vi "PID (DBL) Obsolete.vi"(6 "reinitialize? (F)":bool, 7 "output range":cluster{"output high":dbl, "output low":dbl}={"output high"=100.0, "output low"=-100.0} {"output low" format="%.2f"; "output high" format="%.2f"}, 8 "dt (s)":dbl=-1.0 format="%.3f", 9 "PID gains":T1={"proportional gain (Kc)"=1.0, "integral time (Ti, min)"=0.01, "derivative time (Td, min)"=0.0} {"derivative time (Td, min)" format="%.3f"; "integral time (Ti, min)" format="%.3f"; "proportional gain (Kc)" format="%.3f"}, 10 "process variable":dbl format="%.2f", 11 "setpoint":dbl format="%.2f") -> (0 "dt out (s)":dbl format="%.3f", 3 "output":dbl format="%.2f")   [LabVIEW 2020, in "NI_PID_pid.lvlib"]
doc: "PID algorithm for simple PID applications or high speed control applications that require an efficient algorithm. PID algorithm features control output range limiting with integrator anti-windup and bumpless controller output for PID gain changes."
uses:
  <vilib>/addons/control/pid/NI_PID_pid.lvlib
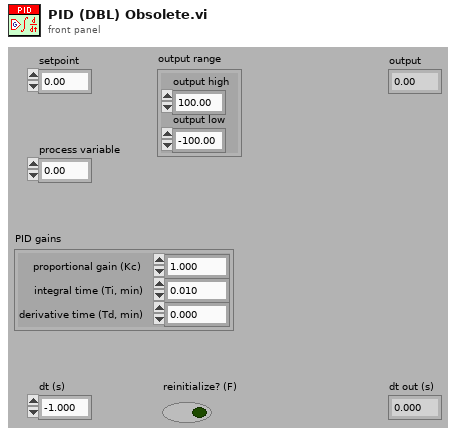
[diagram p1: front panel]
types:
  T1 = cluster{"proportional gain (Kc)":dbl, "integral time (Ti, min)":dbl, "derivative time (Td, min)":dbl}
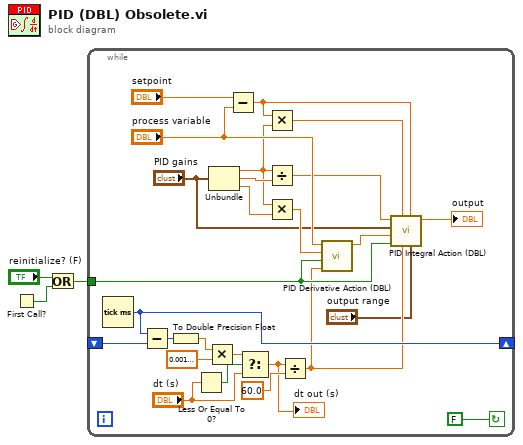
[diagram p0: block diagram]
diagram:
  n1 = First Call?() -> (First Call?: T/F=w3:bool)
  n2 = Or(x="reinitialize? (F)", y=w3) -> (x .or. y?=w2:bool)
  n3 = while {
    tunnel: w2 -> [w9]
    shift-left: _ -> [w23]
    shift-right: [w22] -> _
    stop <- FALSE continue-if-true
    n4 = Tick Count (ms)() -> (millisecond timer value=w22:u32)
    n5 = Subtract(x=w22, y=w23) -> (x-y=w27:u32)
    n6 = To Double Precision Float(number=w27) -> (double precision float=w26:dbl)
    n7 = Less Or Equal To 0?(x="dt (s)") -> (x <= 0?=w24:bool)
    n8 = Multiply(x=w26, y=0.0010000000474974513) -> (x*y=w25:dbl)
    n9 = Unbundle("PID gains") -> ("proportional gain (Kc)"=w15:dbl, "integral time (Ti, min)"=w19:dbl, "derivative time (Td, min)"=w18:dbl)
    n10 = Subtract(x="setpoint", y="process variable") -> (x-y=w12:dbl)
    n11 = Select(t=w25, s=w24, f="dt (s)") -> (s? t:f=w4:dbl)
    "dt out (s)" <- w4
    n12 = Multiply(x=w12, y=w15) -> (x*y=w11:dbl)
    n13 = Divide(x=w15, y=w19) -> (x/y=w13:dbl)
    n14 = Multiply(x=w15, y=w18) -> (x*y=w17:dbl)
    n15 = Divide(x=w4, y=60.0) -> (x/y=w8:dbl)
    n16 = call <vilib>:"PID Derivative Action (DBL).vi"("dt (min)"=w8, "initialize (F)"=w9, "Kd"=w17, "process variable"="process variable") -> ("derivative action"=w10:dbl)  [unwired: 3 out]
    n17 = call <vilib>:"PID Integral Action (DBL).vi"("output range"="output range", "error"=w12, "dt (min)"=w8, "proportional action"=w11, "initialize (F)"=w9, "derivative action"=w10, "PID gains"="PID gains", "Ki"=w13) -> ("output"=→"output":dbl)  [unwired: 3 out]
  }
